vi "CheckIfMove.vi"(0 "Cluster":T1) -> (1 "RawSetPosition":dbl, 2 "RawActPosition":dbl, 3 "Move?":bool)   [LabVIEW 2015, in "CS++SimMotor.lvlib" / "CS++SimMotor.lvclass"]
doc: "This is a small SubVI which checks if the next step for the SimMotor is to move or not."
uses:
  CS++SimMotor.lvclass
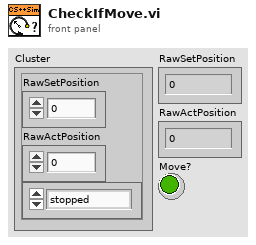
[diagram p1: front panel]
types:
  T1 = cluster{"RawSetPosition":dbl, "RawActPosition":dbl, "Enum":enum16{"stopped", "increasing", "decreasing"}}
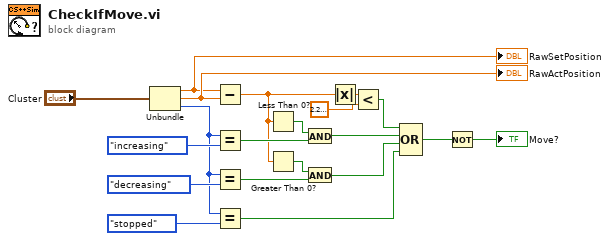
[diagram p0: block diagram]
diagram:
  n1 = Unbundle("Cluster") -> ("RawSetPosition"=w17:dbl, "RawActPosition"=w18:dbl, "Enum"=w3:enum16{"stopped", "increasing", "decreasing"})
  "RawSetPosition" <- w17
  "RawActPosition" <- w18
  n2 = Subtract(x=w17, y=w18) -> (x-y=w8:dbl)
  n3 = Equal?(x=w3, y=enum16{"stopped", "increasing", "decreasing"}."increasing") -> (x = y?=w13:bool)
  n4 = Equal?(x=w3, y=enum16{"stopped", "increasing", "decreasing"}."decreasing") -> (x = y?=w9:bool)
  n5 = Equal?(x=w3, y=enum16{"stopped", "increasing", "decreasing"}."stopped") -> (x = y?=w1:bool)
  n6 = Less Than 0?(x=w8) -> (x < 0?=w12:bool)
  n7 = Greater Than 0?(x=w8) -> (x > 0?=w7:bool)
  n8 = And(x=w12, y=w13) -> (x .and. y?=w11:bool)
  n9 = And(x=w7, y=w9) -> (x .and. y?=w6:bool)
  n10 = Absolute Value(x=w8) -> (abs(x)=w19:dbl)
  n11 = Less?(x=w19, y=2.220446049250313e-16) -> (x < y?=w15:bool)
  n12 = Compound Arithmetic op=OR(w15, w11, w6, w1) -> (w5:bool)
  n13 = Not(x=w5) -> (.not. x?=→"Move?":bool)
